vi "序列号写入.vi"(8 "Error in":errorcluster caption="Error in (no error)", 10 "序列号":string, 11 "MB session in":refnum<class "MB_Master.lvclass">) -> (0 "error out":errorcluster, 3 "MB session out":refnum<class "MB_Master.lvclass">)   [LabVIEW 2016, in "斯坦道总氮.lvlib"]
uses:
  <vilib>/Plasmionique/MB Master/MB_Master/MB_Master.lvclass
  <vilib>/Plasmionique/MB Master/MB Master.lvlib
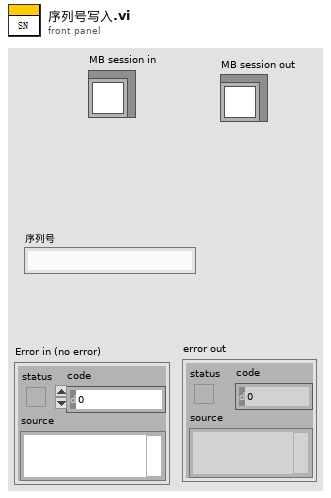
[diagram p1: front panel]
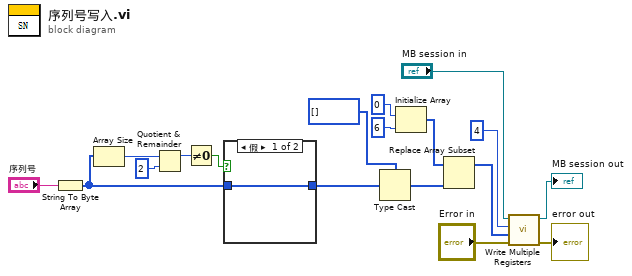
[diagram p0: block diagram]
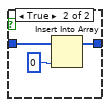
[diagram p2: hidden frame]
diagram:
  n1 = String To Byte Array(string="序列号") -> (unsigned byte array=w4:u8[])
  n2 = Array Size(array=w4) -> (size(s)=w7:i32)
  n3 = Quotient & Remainder(x=w7, y=2) -> (x-y*floor(x/y)=w5:i32)  [unwired: 1 out]
  n4 = Not Equal To 0?(x=w5) -> (x != 0?=w3:bool)
  n5 = case shown="假" w3 {
    tunnel: w4 -> [w19 w22]
    tunnel: [w19 w20] -> w2
    frame False {
    }
    frame True {
      n6 = Insert Into Array(array=w22, new element=u8 0 ("新元素/子数组")) -> (w20:u8[])  [unwired: 1 in]
    }
  }
  n7 = Type Cast(type=u16[] [], x=w2) -> (*(type *) &x=w9:u16[])
  n8 = Initialize Array(u16 0 ("下限"), 6 ("维数大小")) -> (w10:u16[])
  n9 = Replace Array Subset(array=w10, new element=w9) -> (w8:u16[])  [unwired: 1 in]
  n10 = call <vilib>:"Write Multiple Registers.vi"("error in (no error)"="Error in", "values"=w8, "starting address"=u16 4, "MB session in"="MB session in") -> ("error out"=→"error out":errorcluster, "MB session out"=→"MB session out":refnum<class "MB_Master.lvclass">)  [unwired: 6 in]
